vi "counter.vi"(1 "RD":bool, 2 "WR":bool, 3 "R":bool, 4 "C":bool) -> (0 "X":T2)   [LabVIEW 2013]
panel:
  in  "S":T1
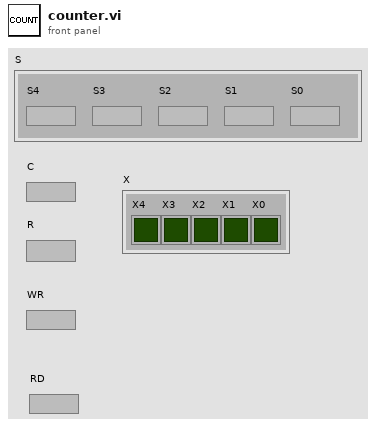
[diagram p1: front panel]
types:
  T1 = cluster{"S4":bool, "S3":bool, "S2":bool, "S1":bool, "S0":bool}
  T2 = cluster{"X4":bool, "X3":bool, "X2":bool, "X1":bool, "X0":bool}
  T3 = cluster{"!Q":bool, "!Q":bool, "!Q":bool, "!Q":bool, "!Q":bool}
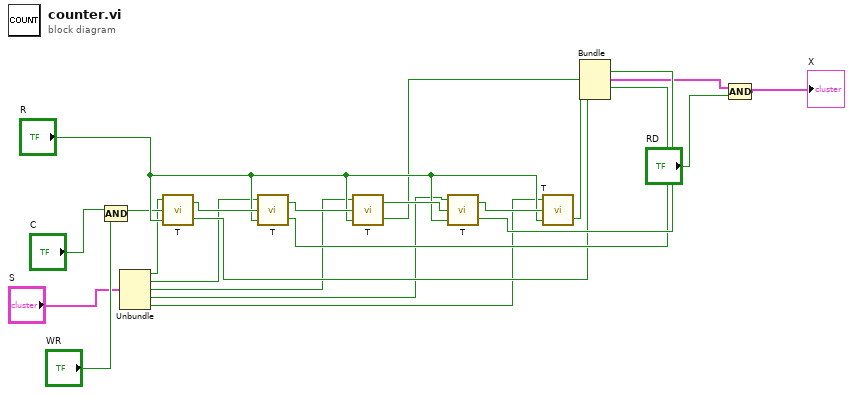
[diagram p0: block diagram]
diagram:
  n1 = Compound Arithmetic op=AND("C", "WR") -> (w12:bool)
  n2 = Unbundle("S") -> ("S4"=w5:bool, "S3"=w4:bool, "S2"=w3:bool, "S1"=w2:bool, "S0"=w1:bool)
  n3 = call "T.vi"("S"="R", "T"=w12, "R"=w5) -> ("!Q"=w13:bool, "Q"=w19:bool)
  n4 = call "T.vi"("S"="R", "T"=w19, "R"=w4) -> ("!Q"=w14:bool, "Q"=w20:bool)
  n5 = call "T.vi"("S"="R", "T"=w20, "R"=w3) -> ("!Q"=w15:bool, "Q"=w21:bool)
  n6 = call "T.vi"("S"="R", "T"=w21, "R"=w2) -> ("!Q"=w16:bool, "Q"=w22:bool)
  n7 = call "T.vi"("S"="R", "T"=w22, "R"=w1) -> ("!Q"=w17:bool)  [unwired: 1 out]
  n8 = Bundle("!Q"=w17, "!Q"=w16, "!Q"=w15, "!Q"=w14, "!Q"=w13) -> (w7:T3)  [unwired: 1 in]
  n9 = Compound Arithmetic op=AND(w7, "RD") -> (→"X":T3)
